vi "Test Log.vi"(8 "error in (no error)":errorcluster, 11 "Post Analysis in":refnum<class "Post Analysis.lvclass">) -> (0 "error out":errorcluster, 3 "Post Analysis out":refnum<class "Post Analysis.lvclass">)   [LabVIEW 2023, in "Data Analysis.lvlib" / "Post Analysis.lvlib" / "Post Analysis.lvclass"]
uses:
  Post Analysis.lvclass
  Post Analysis.lvclass/Post Analysis.ctl
  Data Analysis.lvlib
  HardwareAbstractionLayer_LVOOP/Database/Database.lvclass
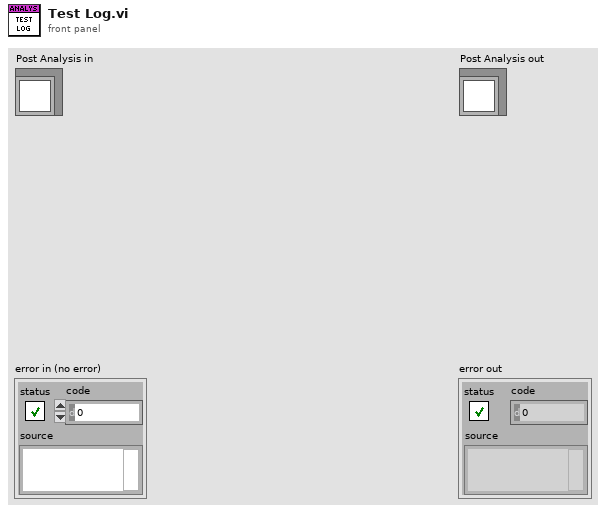
[diagram p1: front panel]
types:
  T1 = cluster{"table":string, "condition":string, "columns":string[]}
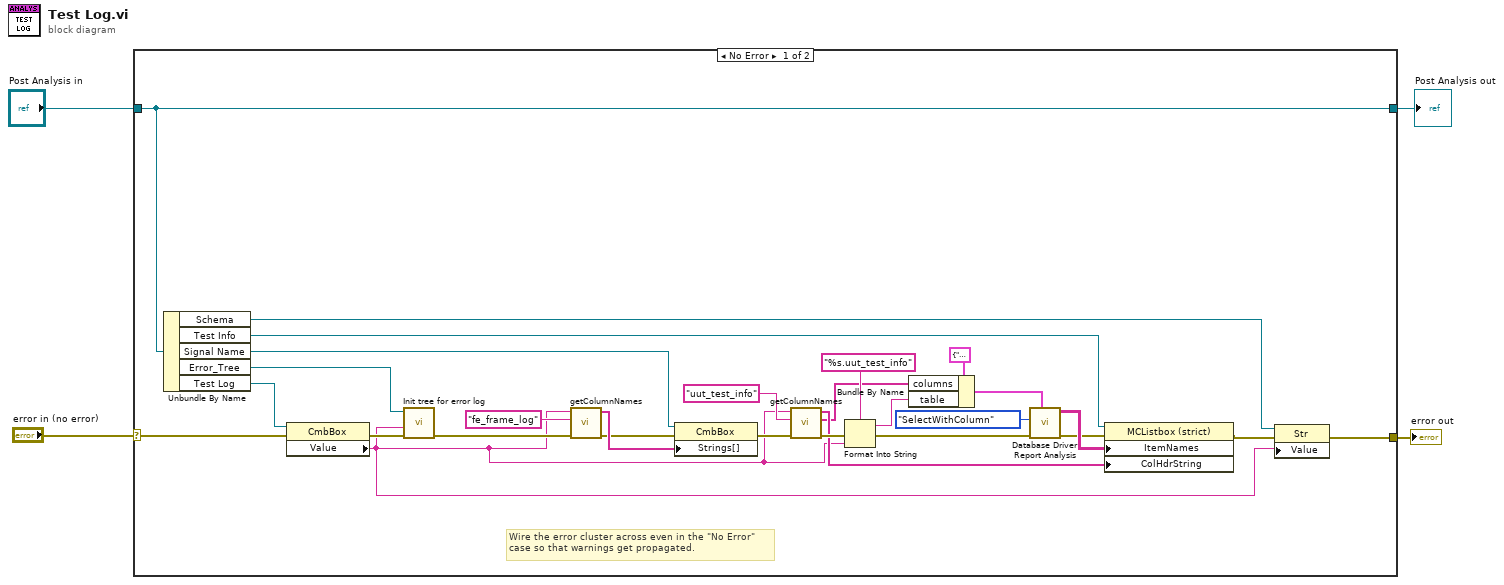
[diagram p0: block diagram]
diagram:
  n1 = case shown="No Error" "error in (no error)" {
    selector: "error in (no error)" -> [w12 w34]
    tunnel: [w5 w34] -> w3
    tunnel: [w15 w33] -> w1
    tunnel: "Post Analysis in" -> [w15 w33]
    frame No Error {
      # "Wire the error cluster across even in the \"No Error\"\ncase so that warnings get propagated."
      n2 = Unbundle By Name(w15) -> ("Schema"=w8:refnum<vi>, "Test Info"=w10:refnum<vi>, "Signal Name"=w9:refnum<vi>, "Error_Tree"=w14:refnum<vi>, "Test Log"=w13:refnum<vi>)
      n3 = property class="CmbBox"(reference=w13, error in=w12) -> (error out=w11:errorcluster, "Value"=w7:string)  [unwired: 1 out]
      n4 = call "Init tree for error log.vi"("error in (no error)"=w11, "Test Log(Schema)"=w7, "TreeControl in"=w14) -> ("error out"=w32:errorcluster)  [unwired: 8 in]
      n5 = call "getColumnNames.vi"("error in (no error)"=w32, "tableName"="fe_frame_log" ("schema"), "schema"=w7) -> ("error out"=w30:errorcluster, "columnNames"=w31:string[])  [unwired: 6 in, 1 out]
      n6 = property on="Property Node" class="CmbBox"(reference=w9, error in=w30, "Strings[]"=w31) -> (error out=w27:errorcluster)  [unwired: 1 out]
      n7 = call "getColumnNames.vi"("error in (no error)"=w27, "tableName"="uut_test_info" ("schema"), "schema"=w7) -> ("error out"=w26:errorcluster, "columnNamesForQuery"=w16:string[], "columnNames"=w17:string[])  [unwired: 6 in]
      n8 = Format Into String(format string="%s.uut_test_info" ("schema"), error in=w26, w7) -> (resulting string=w20:string, error out=w22:errorcluster)  [unwired: 1 in]
      n9 = Bundle By Name(cluster=T1 {"table"="", "condition"="", "columns"=[]} ("SQLTableData"), "columns"=w16, "table"=w20) -> (w19:T1)
      n10 = call "Database Driver Report Analysis.vi"("SQLTableData"=w19, "error in"=w22, "Select"=enum16{"SelectWithQuery", "SelectWithColumn"}."SelectWithColumn") -> ("error out"=w23:errorcluster, "data"=w24:string[][])  [unwired: 5 in, 2 out]
      n11 = property class="MCListbox (strict)"(reference=w10, error in=w23, "ItemNames"=w24, "ColHdrString"=w17) -> (error out=w6:errorcluster)  [unwired: 1 out]
      n12 = property class="Str"(reference=w8, error in=w6, "Value"=w7) -> (error out=w5:errorcluster)  [unwired: 1 out]
    }
    frame Error {
    }
  }
  "error out" <- w3
  "Post Analysis out" <- w1
